vi "Stress Test - Files.vi"() -> ()   [LabVIEW 2016, in "Global_logger.lvlib"]
uses:
  Global_logger.lvlib
  New TSV Logger.vi
panel:
  out "Time per record [s]":dbl
  in  "stop":bool
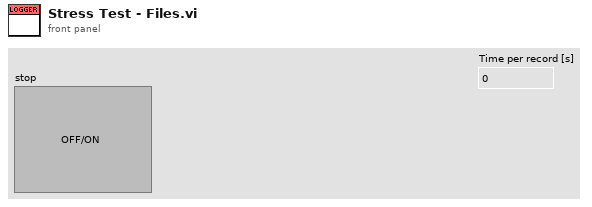
[diagram p1: front panel]
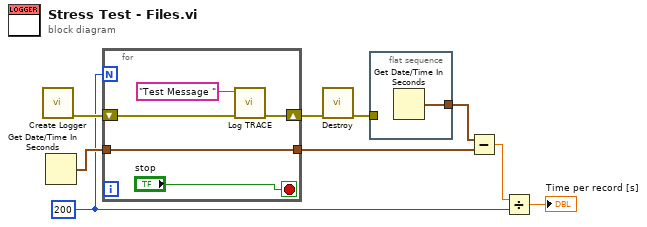
[diagram p0: block diagram]
diagram:
  w1 = 200
  n1 = call-poly "Create Logger.vi"() -> ("error out"=w9:errorcluster)  [unwired: 11 in]
  n2 = Get Date/Time In Seconds() -> (seconds since 1Jan1904=w7:timestamp)
  n3 = for {
    N: w1 -> [_]
    shift-right: [w12] -> w8
    shift-left: w9 -> [w14]
    tunnel: [w10] -> w4
    tunnel: w7 -> [w10]
    stop <- "stop" stop-if-true
    n4 = call "Log TRACE.vi"("error in (no error)"=w14, "Message"="Test Message ") -> ("error out"=w12:errorcluster)  [unwired: 9 in]
  }
  n5 = call "Destroy.vi"("error in (no error)"=w8) -> ("error out"=w6:errorcluster)  [unwired: 10 in]
  n6 = flat-sequence {
    tunnel: w6 -> [_]
    tunnel: [w15] -> w5
    frame #0 {
      n7 = Get Date/Time In Seconds() -> (seconds since 1Jan1904=w15:timestamp)
    }
  }
  n8 = Subtract(x=w5, y=w4) -> (x-y=w3:dbl)
  n9 = Divide(x=w3, y=w1) -> (x/y=→"Time per record [s]":dbl)
